vi "Get requst ID or error.vi"(8 "error in (no error)":errorcluster, 11 "IHandledUnsubscribed in":refnum<class "IHandledUnsubscribed.lvclass">) -> (0 "error out":errorcluster, 1 "ErrorOrSuccess":refnum<class "ErrorOrSuccess.lvclass">, 2 "Unsubscription Request ID":u64, 3 "IHandledUnsubscribed out":refnum<class "IHandledUnsubscribed.lvclass">)   [LabVIEW 2020, in "wamplv.lvlib" / "IHandledUnsubscribed.lvclass"]
uses:
  IHandledUnsubscribed.lvclass
  Message loop classes/ErrorOrSuccess/ErrorOrSuccess.lvclass
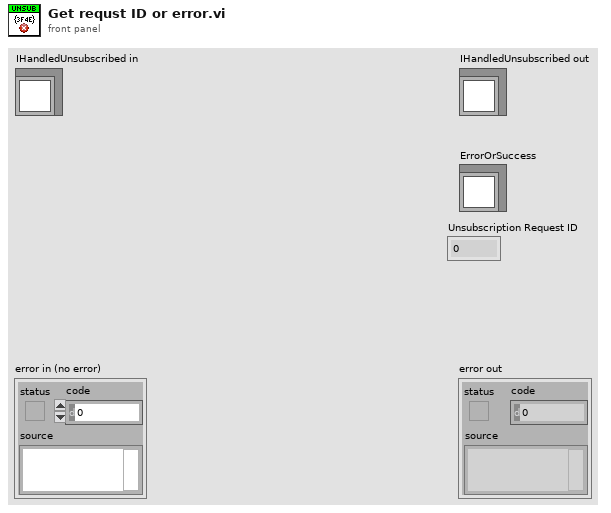
[diagram p1: front panel]
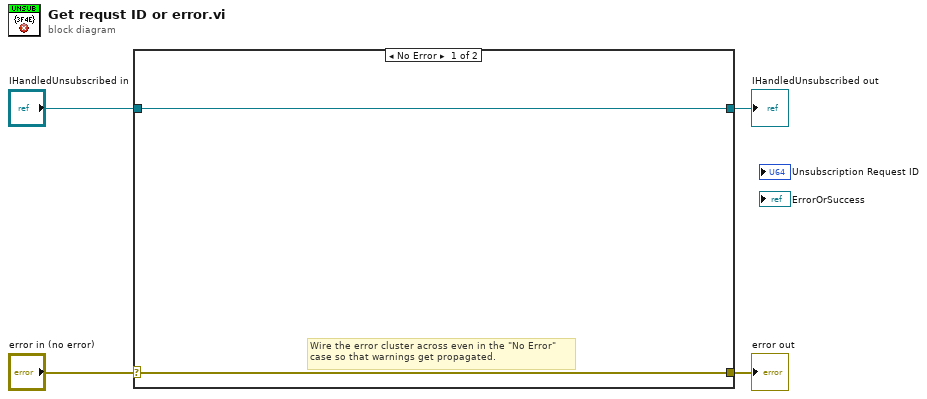
[diagram p0: block diagram]
diagram:
  n1 = case shown="No Error" "error in (no error)" {
    selector: "error in (no error)" -> [w5 w8]
    tunnel: [w5 w8] -> w3
    tunnel: [w6 w7] -> w1
    tunnel: "IHandledUnsubscribed in" -> [w6 w7]
    frame No Error {
      # "Wire the error cluster across even in the \"No Error\"\ncase so that warnings get propagated."
    }
    frame Error {
    }
  }
  "error out" <- w3
  "IHandledUnsubscribed out" <- w1
